vi "(Old Driver) Block Read.vi"(8 "error in (no error)":errorcluster, 9 "Iterations (100)":i32=100, 10 "Channel Counts":i32[](array[numeric])=[1, 10, 100, 1000, 10000, 100000], 11 "VISA resource name":refnum<visa-resource-name>) -> (0 "error out":errorcluster, 1 "Histograms":T1(array[cluster]), 2 "Metrics":T2[](array[typedef]) {"Transfer Rate" format="%.2pB/s"; "Duration Std. Dev." format="%.0f µs"; "Duration Average" format="%.0f µs"}, 3 "VISA resource name out":refnum<visa-resource-name>)   [LabVIEW 2016]
uses:
  Controls/Throughput Metrics.ctl
  <vilib>/Platform/TimedLoop/XDataNode/timing_clust.ctl
  <vilib>/Platform/TimedLoop/XDataNode/nitl_modes.ctl
  <vilib>/Platform/TimedLoop/XDataNode/wakeup.ctl
  <vilib>/platform/TimedLoop/XDataNode/XDataNode.xnode
  <vilib>/Platform/TimedLoop/XDataNode/XDNodeRunTimeDep.lvlib
  <instrlib>/GE 5565 PIORC/GE 5565 PIORC.lvlib
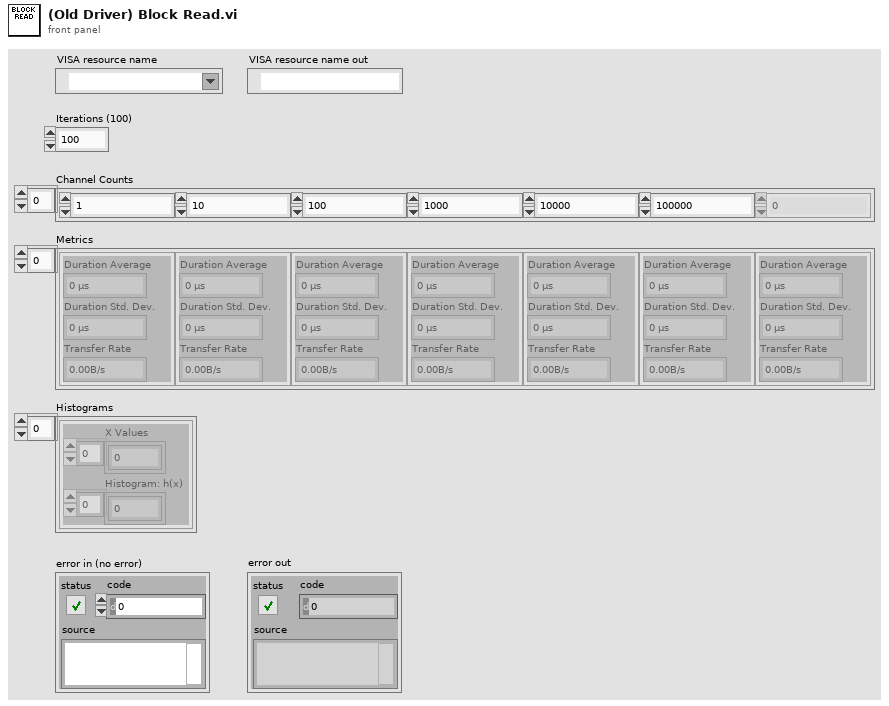
[diagram p1: front panel]
types:
  T1 = cluster{"X Values":dbl[], "Histogram: h(x)":i32[]}[]
  T2 = typedef "Throughput Metrics.ctl" = cluster{"Duration Average":u32, "Duration Std. Dev.":u32, "Transfer Rate":dbl}
  T3 = typedef "XDNodeRunTimeDep.lvlib/timing_clust.ctl" = cluster{"Expected End [f-1]":u64, "Actual End [f-1]":u64, "Finished Late? [f-1]":bool, "Expected End [i-1]":u64, "Actual End [i-1]":u64, "Finished Late? [i-1]":bool, "Expected Start [i]":u64, "Actual Start [i]":u64, "Expected Start [f]":u64, "Actual Start [f]":u64, "Source Name":string, "Structure Name":string, "Period":i64, "Deadline":i64, "Offset":i64, "Start":i64, "Priority":i32, "Timeout":i32, "Mode":T4, "Wakeup Reason":T5, "Error":errorcluster, "Source Type":string, "Secondary Source Type":string, "Global End Time":u64, "Global Start Time":u64, "Frame Duration":u64, "Iteration Duration":u64, "Assigned CPU":i32, "I/O Scan Engine Mode":u32}
  T4 = typedef "XDNodeRunTimeDep.lvlib/nitl_modes.ctl" = enum32{"No Change", "Process missed periods, maintain original phase", "Discard missed periods, maintain original phase", "Process missed periods, ignore original phase", "Discard missed periods, ignore original phase"}
  T5 = typedef "XDNodeRunTimeDep.lvlib/wakeup.ctl" = enum32{"Normal", "Aborted", "Asynchronous wakeup", "Timing source error", "Timed loop error", "Timeout"}
  T6 = cluster{"VMIC 5565 Resource":refnum<visa-resource-name>, "MEMACC Resource":refnum<visa-resource-name>, "byte count":u32, "mem offset":u32}
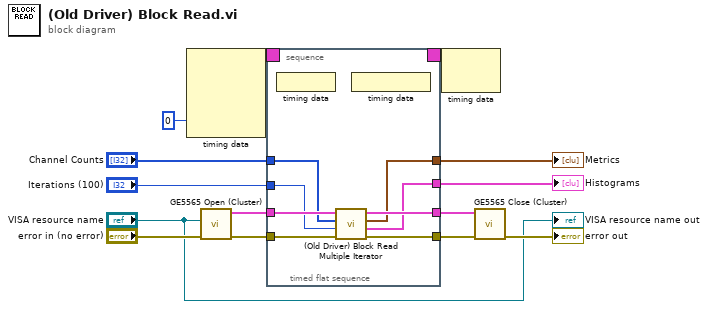
[diagram p0: block diagram]
diagram:
  n1 = node-c288(0 ("Processor")) -> (w14:T3)  [unwired: 3 in]
  n2 = call <instrlib>:"GE5565 Open (Cluster).vi"("error in (no error)"="error in (no error)", "VISA resource name (empty)"="VISA resource name") -> ("error out"=w6:errorcluster, "VMIC-5565"=w5:T6)  [unwired: 4 in]
  n3 = timed-sequence {
    timing: w14 -> [_]
    timing-out: [_] -> w13
    tunnel: w5 -> [w22]
    tunnel: w6 -> [w21]
    tunnel: [w20] -> w3
    tunnel: [w19] -> w4
    tunnel: "Iterations (100)" -> [w18]
    tunnel: "Channel Counts" -> [w17]
    tunnel: [w16] -> w9
    tunnel: [w15] -> w8
    n4 = timed-flat-sequence {
      tunnel: w22 -> [w30]
      tunnel: w21 -> [w29]
      tunnel: [w27] -> w20
      tunnel: [w28] -> w19
      tunnel: w18 -> [w26]
      tunnel: w17 -> [w25]
      tunnel: [w24] -> w16
      tunnel: [w23] -> w15
      n5 = node-c288() -> ()  [unwired: 1 in]
      n6 = call "(Old Driver) Block Read Multiple Iterator.vi"("error in (no error)"=w29, "Iterations (1000)"=w26, "Channel Counts"=w25, "VMIC-5565"=w30) -> ("error out"=w27:errorcluster, "Histograms"=w23:T1, "Metrics"=w24:T2[], "VMIC-5565 out"=w28:T6)  [unwired: 4 in]
      n7 = node-c288() -> ()  [unwired: 1 out]
    }
  }
  "Metrics" <- w9
  "Histograms" <- w8
  n8 = node-c288(w13) -> ()  [unwired: 1 out]
  n9 = call <instrlib>:"GE5565 Close (Cluster).vi"("error in (no error)"=w3, "VMIC reference in"=w4) -> ("error out"=→"error out":errorcluster)  [unwired: 5 in]
  "VISA resource name out" <- "VISA resource name"
